vi "GetFlattenedString.vi"(8 "error in":errorcluster, 11 "UnsignedByte in":refnum<class "UnsignedByte.lvclass">) -> (0 "error out":errorcluster, 2 "FlattenedString":string, 3 "UnsignedByte out":refnum<class "UnsignedByte.lvclass">)   [LabVIEW 2021, in "ProligentXMLGenerator.lvlib" / "UnsignedByte.lvclass"]
uses:
  UnsignedByte.lvclass
  UnsignedByte.lvclass/UnsignedByte.ctl
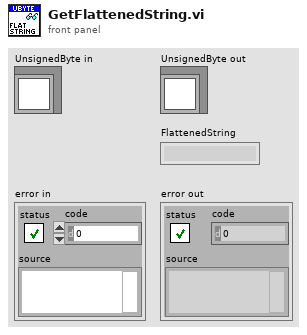
[diagram p1: front panel]
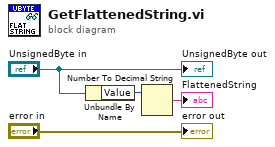
[diagram p0: block diagram]
diagram:
  n1 = Unbundle By Name("UnsignedByte in") -> ("Value"=w2:u8)
  n2 = Number To Decimal String(number=w2) -> (decimal integer string=→"FlattenedString":string)  [unwired: 1 in]
  "error out" <- "error in"
  "UnsignedByte out" <- "UnsignedByte in"
